vi "Write Mode.vi"(8 "Error In":errorcluster, 10 "Mode":T1 items=["Non-Blocking", "Blocking"], 11 "Channel In":refnum<class "Channel.lvclass">) -> (0 "Error Out":errorcluster, 3 "Channel Out":refnum<class "Channel.lvclass">)   [LabVIEW 2018, in "Toolkit.lvlib" / "Channel.lvclass"]
doc: "Sets the type communication for this channel."
uses:
  Channel.lvclass
  Type Definitions/Modes.ctl
  Channel.lvclass/Channel.ctl
  Session/Session.lvclass/Session.ctl
  SSH/SSH.lvclass/SSH.ctl
  Session/Session.lvclass
  Toolkit.lvlib
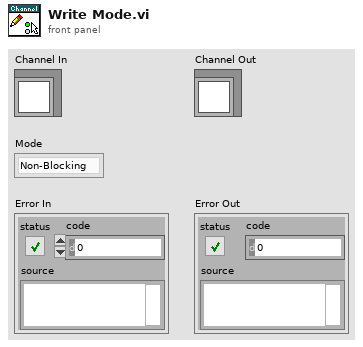
[diagram p1: front panel]
types:
  T1 = typedef "Toolkit.lvlib/Channel.lvclass/Modes.ctl" = i32
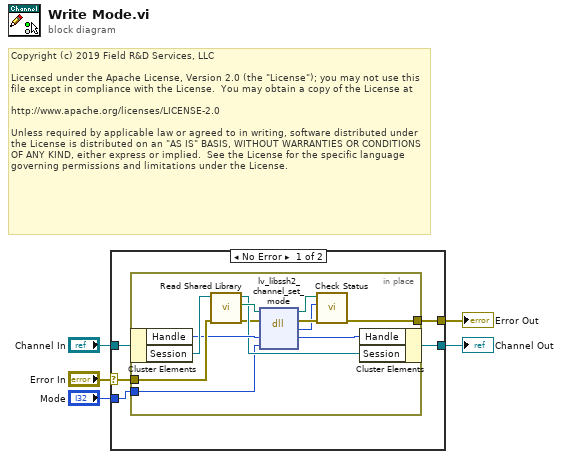
[diagram p0: block diagram]
diagram:
  # "Copyright (c) 2019 Field R&D Services, LLC\n\nLicensed under the Apache License, Version 2.0 (the \"License\"); you may not use this file except in compliance with the License.  You may obtain a copy of the License at\n\nhttp://www.apache.org/licenses/LICENSE-2.0\n\nUnless required by applicable law or agreed to in writing, software distributed under the License is distributed on an \"AS IS\" BASIS, WITHOUT WARRANTIES OR CONDITIONS OF ANY KIND, either express or implied.  See the License for the specific language governing permissions and limitations under the License."
  n1 = case shown="No Error" "Error In" {
    selector: "Error In" -> [w8 w24]
    tunnel: [w7 w24] -> w4
    tunnel: "Channel In" -> [w10 w23]
    tunnel: [w9 w23] -> w2
    tunnel: "Mode" -> [w6 _]
    frame No Error {
      n2 = in-place {
        in-place-border: w8 -> [w20]
        in-place-border: [w16] -> w7
        in-place-border: w6 -> [w11]
        n3 = in-place-cluster #1(w10) -> ("Handle"=w15:u64, "Session"=w22:refnum<class "Session.lvclass">)
        n4 = call "Read Shared Library.vi"("Error In"=w20, "Session In"=w22) -> ("Erorr Out"=w12:errorcluster, "libssh2lv Shared Library"=w21:path, "Session Out"=w13:refnum<class "Session.lvclass">)  [unwired: 7 in]
        n5 = dll-call lib="libssh2lv.*" fn="lv_libssh2_channel_set_mode"(path in=w21, error in=w12, "handle"=w15, "mode"=w11) -> (path out=w18:path, error out=w19:errorcluster, "status"=w17:i32, "handle"=w14:u64)  [unwired: 2 in]
        n6 = call "Check Status.vi"("Error In"=w19, "Status"=w17, "libssh2lv Shared Library In"=w18) -> ("Error Out"=w16:errorcluster)  [unwired: 7 in, 1 out]
        n7 = in-place-cluster #1("Handle"=w14, "Session"=w13) -> (w9:refnum<class "Channel.lvclass">)
      }
    }
    frame Error {
    }
  }
  "Error Out" <- w4
  "Channel Out" <- w2
